vi "LESO_close.vi"(8 "error in (no error)":errorcluster, 11 "Handle in":u32) -> (0 "error out":errorcluster, 2 "FT_Status":u32)   [LabVIEW 2012]
doc: "Закрывает устройство. Освобождает Handle."
uses:
  FTD2XX.dll
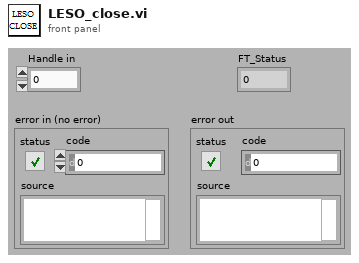
[diagram p1: front panel]
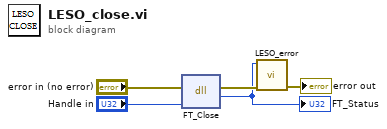
[diagram p0: block diagram]
diagram:
  n1 = dll-call lib="FTD2XX.dll" fn="FT_Close"(error in="error in (no error)", "Handle"="Handle in") -> (error out=w4:errorcluster, "FT_Status"=w3:u32)  [unwired: 3 in, 1 out]
  "FT_Status" <- w3
  n2 = call "LESO_error.vi"("error in"=w4, "FT_Status"=w3) -> ("error out"=→"error out":errorcluster)  [unwired: 9 in]
